vi "RMS PtByPt.vi"(2 "initialize":bool, 3 "sample length":i32=100, 5 "x":dbl format="%0.2f") -> (0 "error":i32, 1 "rms value":dbl format="%0.2f")   [LabVIEW 2020, in "NI_PtbyPt.lvlib"]
doc: "Computes the root mean square (rms) of the set of input data points specified by <B>sample length</B>."
uses:
  NI_PtbyPt.lvlib
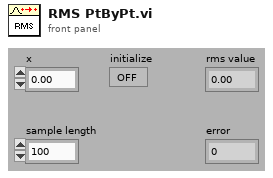
[diagram p1: front panel]
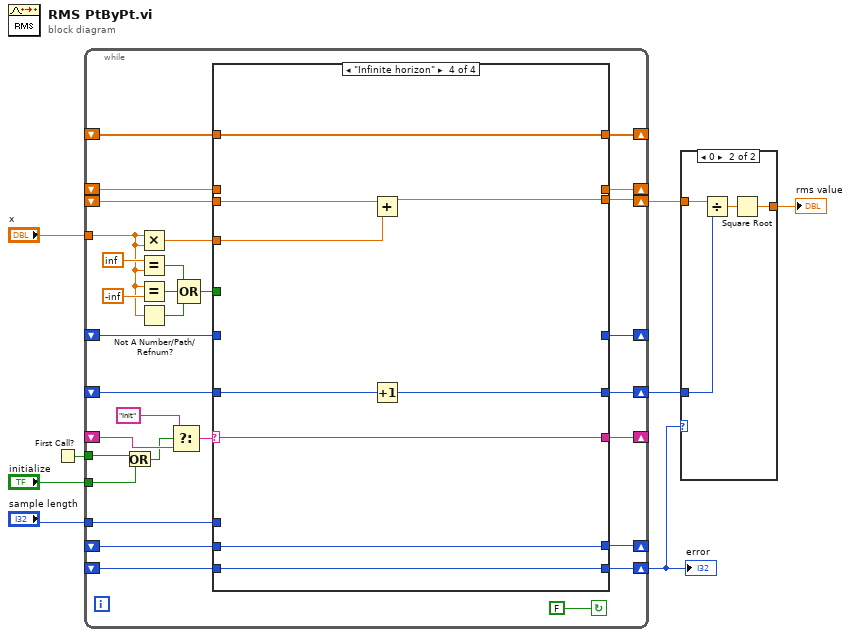
[diagram p0: block diagram]
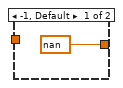
[diagram p2: hidden frame]
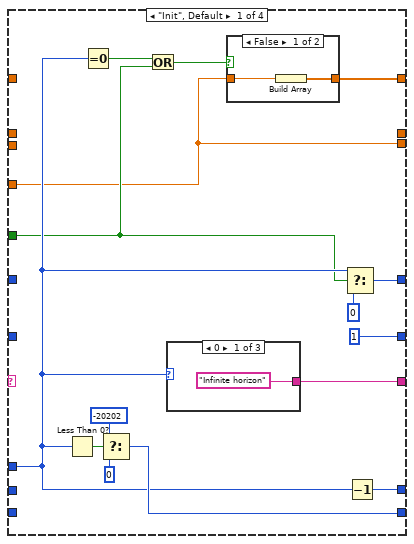
[diagram p3: hidden frame]
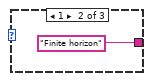
[diagram p5: hidden frame]
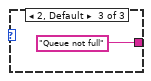
[diagram p6: hidden frame]
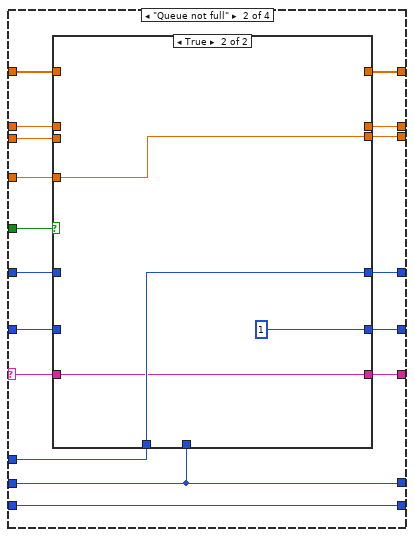
[diagram p7: hidden frame]
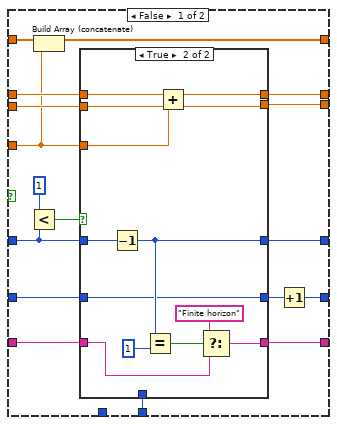
[diagram p8: hidden frame]
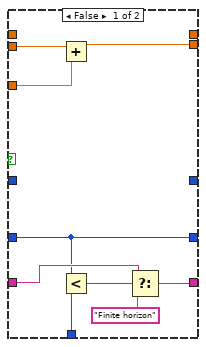
[diagram p9: hidden frame]
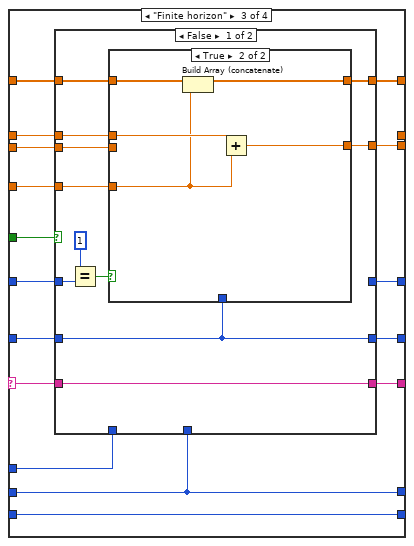
[diagram p10: hidden frame]
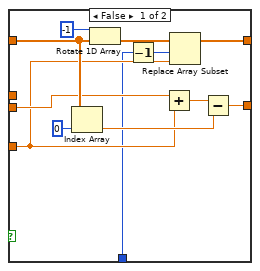
[diagram p11: hidden frame]
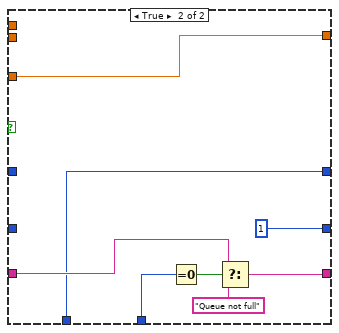
[diagram p12: hidden frame]
diagram:
  n1 = First Call?() -> (First Call?: T/F=w5:bool)
  n2 = while {
    tunnel: w5 -> [w26]
    shift-left: _ -> [w28]
    shift-right: [w29] -> _
    shift-left: _ -> [w30]
    shift-right: [w31] -> w8
    shift-left: _ -> [w33]
    shift-right: [w32] -> _
    shift-left: _ -> [w35]
    shift-right: [w36] -> w7
    shift-left: _ -> [w39]
    shift-right: [w34] -> _
    shift-right: [w18] -> _
    shift-left: _ -> [w17]
    shift-right: [w16] -> _
    shift-left: _ -> [w15]
    shift-right: [w13] -> w4
    shift-left: _ -> [w12]
    tunnel: "x" -> [w11]
    tunnel: "sample length" -> [w10]
    tunnel: "initialize" -> [w9]
    stop <- FALSE continue-if-true
    n3 = Or(x=w26, y=w9) -> (x .or. y?=w25:bool)
    n4 = Multiply(x=w11, y=w11) -> (x*y=w14:dbl)
    n5 = Equal?(x=inf, y=w11) -> (x = y?=w21:bool)
    n6 = Equal?(x=w11, y=-inf) -> (x = y?=w22:bool)
    n7 = Not A Number/Path/Refnum?(number/path/refnum=w11) -> (NaN/Path/Refnum?=w20:bool)
    n8 = Select(t="Init", s=w25, f=w39) -> (s? t:f=w37:string)
    n9 = Compound Arithmetic op=OR(w21, w22, w20) -> (w19:bool)
    n10 = case shown="\"Infinite horizon\"" w37 {
      selector: w37 -> [_ w72 w129 w178]
      tunnel: w14 -> [w40 w61 w120 w173]
      tunnel: [1 w74 w127 w171] -> w36
      tunnel: w35 -> [_ w73 w134 w179]
      tunnel: [w46 w71 w128 w178] -> w34
      tunnel: w33 -> [_ w76 w132 w177]
      tunnel: [w41 w75 w133 w177] -> w32
      tunnel: w10 -> [w45 w63 w122 _]
      tunnel: [w40 w70 w130 w175] -> w31
      tunnel: w30 -> [_ w69 w131 w176]
      tunnel: [w50 w68 w123 w174] -> w29
      tunnel: w28 -> [_ w68 w123 w174]
      tunnel: w19 -> [w43 w67 w126 _]
      tunnel: [w48 w62 w121 _] -> w18
      tunnel: w17 -> [_ w66 w125 _]
      tunnel: [_ w65 _ _] -> w16
      tunnel: w15 -> [_ w64 w124 _]
      tunnel: [w47 w60 w119 w172] -> w13
      tunnel: w12 -> [_ w60 w119 w172]
      frame "Init", Default {
        n11 = Less Than 0?(x=w45) -> (x < 0?=w51:bool)
        n12 = Equal To 0?(x=w45) -> (x = 0?=w44:bool)
        n13 = Select(t=-20202, s=w51, f=0) -> (s? t:f=w47:i32)
        n14 = Or(x=w44, y=w43) -> (x .or. y?=w42:bool)
        n15 = case shown="0" w45 {
          tunnel: ["Infinite horizon" "Finite horizon" "Queue not full" ("f")] -> w46
          frame 0 {
          }
          frame 1 {
          }
          frame 2, Default {
          }
        }
        n16 = case shown="False" w42 {
          tunnel: [w56 _] -> w41
          tunnel: w40 -> [w55 _]
          frame False {
            n17 = Build Array(w55) -> (w56:dbl[])
          }
          frame True {
          }
        }
        n18 = Select(t=w45, s=w43, f=0) -> (s? t:f=w48:i32)
        n19 = Decrement(x=w45) -> (x-1=w50:i32)
      }
      frame "Queue not full" {
        n20 = case shown="True" w67 {
          tunnel: w76 -> [w93 _]
          tunnel: [w92 _] -> w75
          tunnel: [w85 1] -> w74
          tunnel: w73 -> [w91 _]
          tunnel: w72 -> [w90 w116]
          tunnel: [w89 w116] -> w71
          tunnel: [w88 w117] -> w70
          tunnel: w69 -> [w87 _]
          tunnel: w61 -> [w79 w117]
          tunnel: w68 -> [w86 _]
          tunnel: w66 -> [w78 _]
          tunnel: [w81 _] -> w65
          tunnel: w64 -> [w80 _]
          tunnel: w63 -> [_ w118]
          tunnel: [w77 w118] -> w62
          frame False {
            n21 = Less?(x=1, y=w78) -> (x < y?=w82:bool)
            n22 = Build Array (concatenate)(w93, w79) -> (w92:dbl[])
            n23 = case shown="True" w82 {
              tunnel: w91 -> [w95 w103]
              tunnel: w90 -> [w101 w108]
              tunnel: [w99 w109] -> w89
              tunnel: [w98 w107] -> w88
              tunnel: w87 -> [w97 w107]
              tunnel: w86 -> [w96 _]
              tunnel: [w95 w103] -> w84
              tunnel: [_ w114] -> w81
              tunnel: w79 -> [w94 w106]
              tunnel: w80 -> [_ w113]
              tunnel: w78 -> [_ w105]
              tunnel: [_ w104] -> w77
              frame False {
                n24 = Add(x=w97, y=w94) -> (x+y=w98:dbl)
                n25 = Less?(x=w95, y=w96) -> (x < y?=w102:bool)
                n26 = Select(t=w101, s=w102, f="Finite horizon") -> (s? t:f=w99:string)
              }
              frame True {
                n27 = Decrement(x=w105) -> (x-1=w104:i32)
                n28 = Equal?(x=w104, y=1) -> (x = y?=w112:bool)
                n29 = Add(x=w113, y=w106) -> (x+y=w114:dbl)
                n30 = Select(t="Finite horizon" ("f"), s=w112, f=w108) -> (s? t:f=w109:string)
              }
            }
            n31 = Increment(x=w84) -> (x+1=w85:i32)
          }
          frame True {
          }
        }
      }
      frame "Finite horizon" {
        n32 = case shown="False" w126 {
          tunnel: w134 -> [w139 _]
          tunnel: [w145 _] -> w133
          tunnel: w132 -> [w144 _]
          tunnel: w131 -> [w143 _]
          tunnel: [w142 w170] -> w130
          tunnel: w120 -> [w141 w170]
          tunnel: w129 -> [w140 w165]
          tunnel: [w140 w167] -> w128
          tunnel: [w139 1] -> w127
          tunnel: w125 -> [w137 _]
          tunnel: w124 -> [w135 _]
          tunnel: w123 -> [_ w166]
          tunnel: w122 -> [_ w163]
          tunnel: [_ w163] -> w121
          frame False {
            n33 = Equal?(x=1, y=w137) -> (x = y?=w136:bool)
            n34 = case shown="True" w136 {
              tunnel: [w153 w158] -> w145
              tunnel: w144 -> [w152 w160]
              tunnel: w143 -> [w151 _]
              tunnel: [w149 w161] -> w142
              tunnel: w141 -> [w147 w159]
              tunnel: w139 -> [w146 _]
              tunnel: w135 -> [_ w162]
              frame False {
                n35 = Index Array(array=w152, index=0 ("Index")) -> (element=w148:dbl)
                n36 = Rotate 1D Array(1:w152, 2:i16 -1 ("n")) -> (0:w155:dbl[])
                n37 = Decrement(x=w146) -> (x-1=w154:i32)
                n38 = Add(x=w151, y=w147) -> (x+y=w150:dbl)
                n39 = Replace Array Subset(array=w155, new element=w147, index=w154) -> (w153:dbl[])
                n40 = Subtract(x=w150, y=w148) -> (x-y=w149:dbl)
              }
              frame True {
                n41 = Build Array (concatenate)(w160, w159) -> (w158:dbl[])
                n42 = Add(x=w162, y=w159) -> (x+y=w161:dbl)
              }
            }
          }
          frame True {
            n43 = Equal To 0?(x=w166) -> (x = 0?=w169:bool)
            n44 = Select(t=w165, s=w169, f="Queue not full") -> (s? t:f=w167:string)
          }
        }
      }
      frame "Infinite horizon" {
        n45 = Add(x=w176, y=w173) -> (x+y=w175:dbl)
        n46 = Increment(x=w179) -> (x+1=w171:i32)
      }
    }
  }
  "error" <- w4
  n47 = case shown="0" w4 {
    tunnel: w8 -> [_ w184]
    tunnel: w7 -> [_ w183]
    tunnel: [nan w181] -> w6
    frame -1, Default {
    }
    frame 0 {
      n48 = Divide(x=w184, y=w183) -> (x/y=w182:dbl)
      n49 = Square Root(x=w182) -> (sqrt(x)=w181:dbl)
    }
  }
  "rms value" <- w6
